vi "Ejemplo llamada.vi"() -> ()   [LabVIEW 2019]
uses:
  Libraries/FunctionGenerator/FunctionGenerator.lvlib
  <vilib>/PantherLAB/FingerPrintReader/Libraries/USBFingerPrintReader/PantherLAB_lib_USBFingerPrintReader.lvlib
panel:
  out "Waveform Graph":waveform(dbl)(graph)
  in  "signal type":T1(ring)
  in  "Offset":dbl
  in  "Frecuency":dbl
  in  "Amplitude":dbl
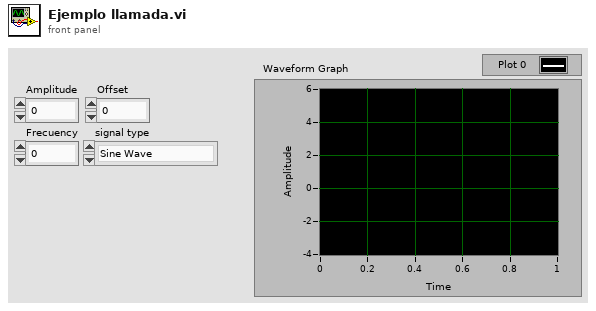
[diagram p1: front panel]
types:
  T1 = enum16{"Sine Wave", "Triangle Wave", "Square Wave", "Sawtooth Wave"}
  T2 = typedef "FunctionGenerator.lvlib/Broadcast Events--cluster.ctl" = cluster{"Module Did Init":refnum<user-event>, "Status Updated":refnum<user-event>, "Error Reported":refnum<user-event>, "Module Did Stop":refnum<user-event>, "Update Module Execution Status":refnum<user-event>, "Waveform Acquired":refnum<user-event>}
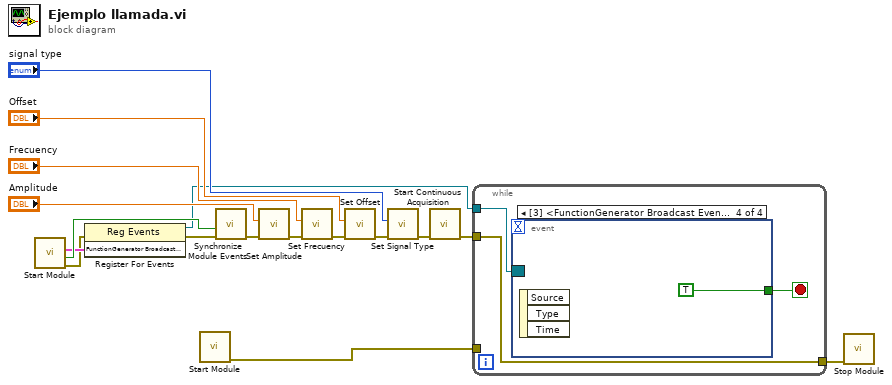
[diagram p0: block diagram]
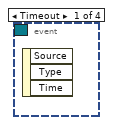
[diagram p2: hidden frame]
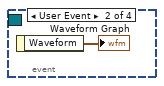
[diagram p3: hidden frame]
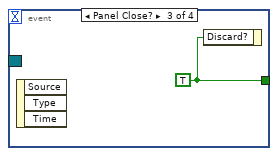
[diagram p4: hidden frame]
diagram:
  n1 = call <vilib>:"Start Module.vi"() -> ("error out"=w6:errorcluster, "Wait for Event Sync?"=w13:bool, "FunctionGenerator Broadcast Events"=w8:T2)  [unwired: 7 in, 2 out]
  n2 = register-events(error in=w6, w8) -> (reference out=w7:refnum<event-registration>, error out=w5:errorcluster)  [unwired: 1 in]
  n3 = call <vilib>:"Start Module.vi"() -> ("error out"=w1:errorcluster)  [unwired: 7 in, 4 out]
  n4 = call "Synchronize Module Events.vi"("error in"=w5, "Wait for Event Sync?"=w13) -> ("error out"=w16:errorcluster)  [unwired: 9 in]
  n5 = call "Set Amplitude.vi"("error in"=w16, "Amplitude"="Amplitude") -> ("error out"=w15:errorcluster)  [unwired: 9 in]
  n6 = call "Set Frecuency.vi"("error in"=w15, "Frecuency"="Frecuency") -> ("error out"=w14:errorcluster)  [unwired: 9 in]
  n7 = call "Set Offset.vi"("error in"=w14, "Offset"="Offset") -> ("error out"=w17:errorcluster)  [unwired: 9 in]
  n8 = call "Set Signal Type.vi"("error in"=w17, "signal type"="signal type") -> ("error out"=w4:errorcluster)  [unwired: 9 in]
  n9 = call "Start Continuous Acquisition.vi"("error in"=w4) -> ("error out"=w3:errorcluster)  [unwired: 10 in]
  n10 = while {
    tunnel: w7 -> [w20]
    tunnel: w3 -> [w18]
    tunnel: [w18] -> w2
    tunnel: w1 -> [_]
    stop <- w19 stop-if-true
    n11 = event shown="[3] <FunctionGenerator Broadcast Events.Module Did Stop>: User Event" {
      selector: w20 -> [_ _ _ _]
      dyn-events: _ -> [_ _ _ _]
      timeout: _ -> [_ _ _ _]
      tunnel: [_ _ w22 TRUE ("Discard?")] -> w19
      event Timeout {
        n12 = event-data() -> ()  [unwired: 1 in, 3 out]
      }
      event User Event {
        n13 = event-data() -> ("Waveform"=→"Waveform Graph":waveform(dbl))  [unwired: 1 in]
      }
      event Panel Close? {
        w22 = TRUE ("Discard?")
        n14 = event-data() -> ()  [unwired: 1 in, 3 out]
        n15 = event-data("Discard?"=w22) -> ()  [unwired: 1 in, 1 out]
      }
      event User Event {
        n16 = event-data() -> ()  [unwired: 1 in, 3 out]
      }
    }
  }
  n17 = call "Stop Module.vi"("error in"=w2) -> ()  [unwired: 10 in, 1 out]
